vi "DefensePsSkill.vi"(9 "Game in":refnum<class "Game.lvclass">, 10 "Robot":refnum<class "Robot.lvclass">, 11 "DefensePsSkill in":refnum<class "DefensePsSkill.lvclass">) -> (2 "Robot out":refnum<class "Robot.lvclass">, 3 "DefensePsSkill out":refnum<class "DefensePsSkill.lvclass">)   [LabVIEW 2023, in "DefensePsSkill.lvclass"]
uses:
  DefensePsSkill.lvclass
  Robot_class/Robot.lvclass
  Game_class/Game.lvclass
panel:
  out "error out 2":errorcluster
  in  "error in (no error) 2":errorcluster
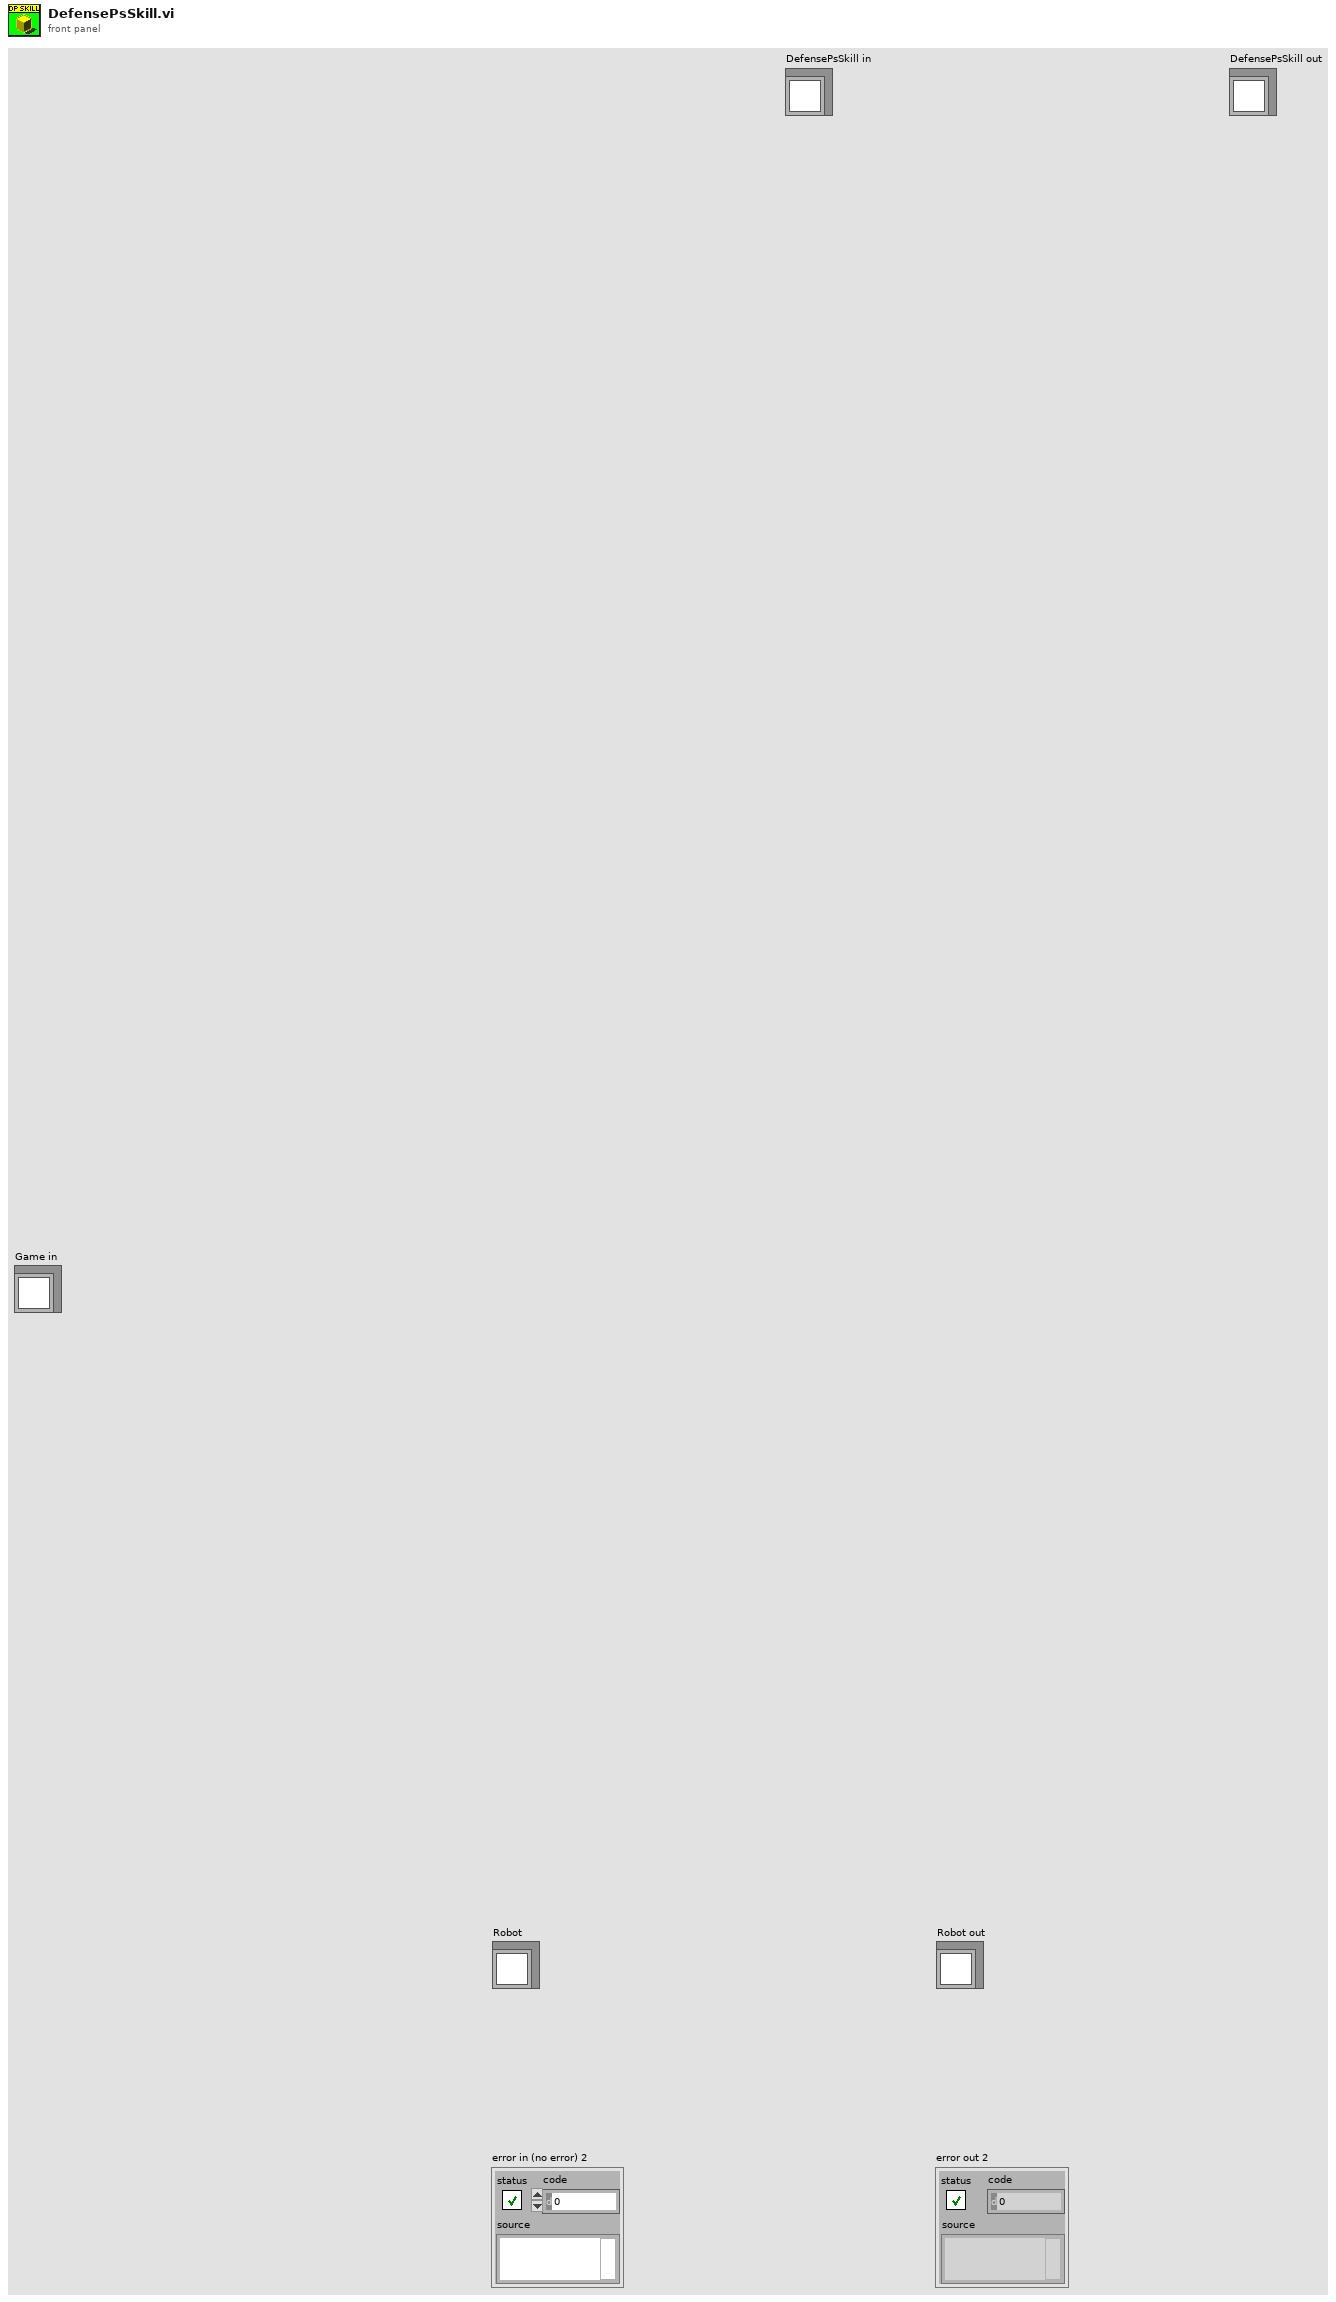
[diagram p1: front panel]
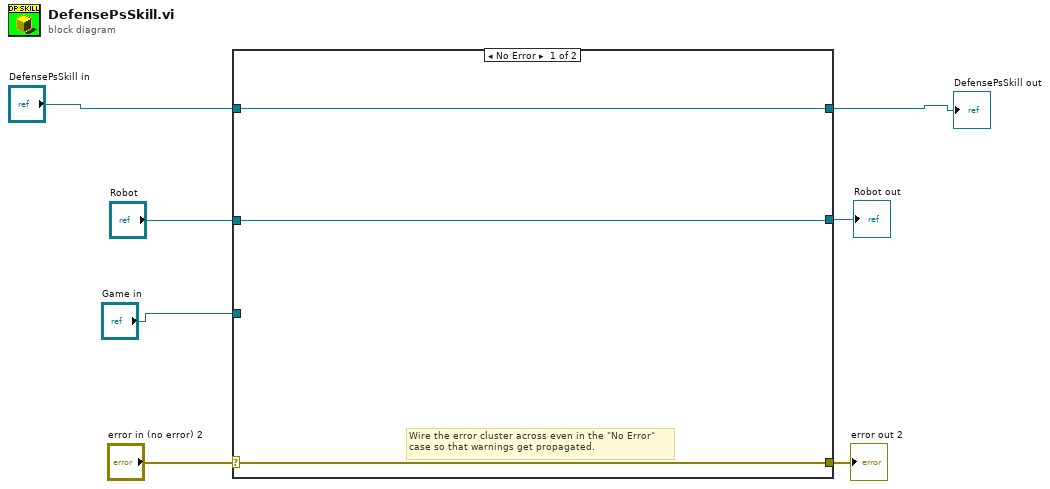
[diagram p0: block diagram]
diagram:
  n1 = case shown="No Error" "error in (no error) 2" {
    selector: "error in (no error) 2" -> [w9 w13]
    tunnel: [w9 w13] -> w6
    tunnel: [w10 w12] -> w2
    tunnel: "DefensePsSkill in" -> [w10 w12]
    tunnel: "Robot" -> [w8 w11]
    tunnel: [w8 w11] -> w4
    tunnel: "Game in" -> [_ _]
    frame No Error {
      # "Wire the error cluster across even in the \"No Error\"\ncase so that warnings get propagated."
    }
    frame Error {
    }
  }
  "DefensePsSkill out" <- w2
  "error out 2" <- w6
  "Robot out" <- w4
